vi "Get Magnet Field.vi"(6 "Axis":T1, 8 "error in (no error)":errorcluster, 11 "Instrument.Oxford1820 in":refnum<class "Instrument.OxfordVRM.lvclass">) -> (0 "error out":errorcluster, 1 "Status":variant, 2 "B Field (T)":dbl, 3 "Instrument.Oxford1820 out":refnum<class "Instrument.OxfordVRM.lvclass">, 4 "Finished?":bool)   [LabVIEW 2016, in "Instrument.OxfordVRM.lvclass"]
uses:
  Instrument.OxfordVRM.lvclass
  <userlib>/LevyLab/Levylab Instruments/Instrument Types/Cryostat/Typedefs/Magnet Axis--Enum.ctl
  <userlib>/LevyLab/postgreSQL-timescaleDB/Data.PG/API/Read Variable (double).vi
  <userlib>/LevyLab/postgreSQL-timescaleDB/Data.PG/API/Read Variable (string).vi
  <userlib>/LevyLab/postgreSQL-timescaleDB/Data.PG/Data.PGSQL.lvclass
  <userlib>/LevyLab/Levylab Instruments/Instrument Types/Cryostat/Instrument.Cryostat.lvclass
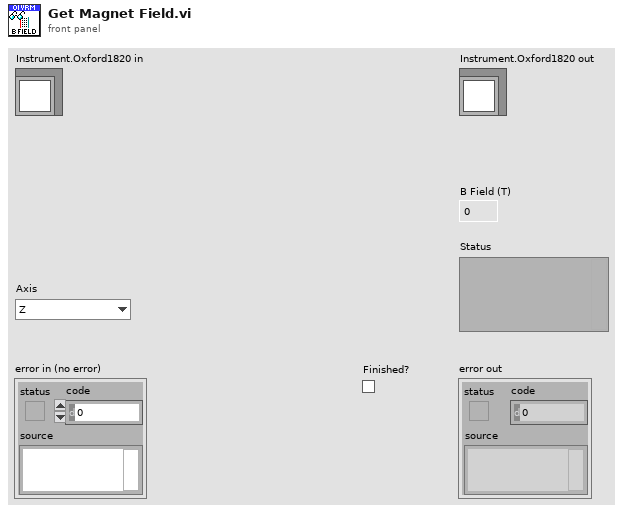
[diagram p1: front panel]
types:
  T1 = typedef "Instrument.Cryostat.lvclass/Magnet Axis--Enum.ctl" = enum16{"Z", "X", "Y"}
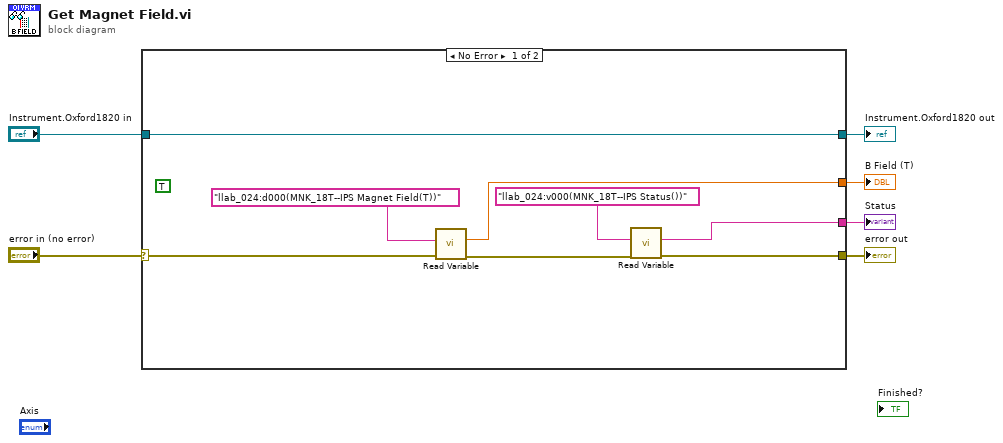
[diagram p0: block diagram]
diagram:
  n1 = case shown="No Error" "error in (no error)" {
    selector: "error in (no error)" -> [w13 w16]
    tunnel: "Instrument.Oxford1820 in" -> [w11 w15]
    tunnel: [w11 w15] -> w5
    tunnel: [w14 _] -> w4
    tunnel: [w12 w16] -> w2
    tunnel: [w10 _] -> w1
    frame No Error {
      (unwired) TRUE
      n2 = call-poly <userlib>:"Read Variable.vi"("error in (no error)"=w13, "PG path"="llab_024:d000(MNK_18T--IPS Magnet Field(T))") -> ("error out"=w9:errorcluster, "Value"=w14:dbl)  [unwired: 4 in, 4 out]
      n3 = call-poly <userlib>:"Read Variable.vi"("error in (no error)"=w9, "PG path"="llab_024:v000(MNK_18T--IPS Status())") -> ("error out"=w12:errorcluster, "Value"=w10:string)  [unwired: 4 in, 4 out]
    }
    frame Error {
    }
  }
  "error out" <- w2
  "Instrument.Oxford1820 out" <- w5
  "B Field (T)" <- w4
  "Status" <- w1
